vi "Protocol.Output Messages.vi"(8 "error in (no error)":errorcluster, 11 "J1939 Main Configuration":T1 {"Stream Refs"."Port Settings"."FD ISO Mode" items=["ISO", "Non ISO", "ISO Legacy"]; "Stream Refs"."Port Settings"."Termination" items=["Off", "On"]; "Stream Refs"."Port Settings"."Mode" items=["CAN 2.0", "CAN FD", "CAN FD+BRS"]}) -> (0 "error out":errorcluster)   [LabVIEW 2023, in "J1939 Addon Engine.lvlib"]
uses:
  J1939 Addon Engine.lvlib
  Types/Protocol.Configuration.ctl
  <vilib>/NI/NI VeriStand Addon Network Comm/Engine/VeriStand Comm.lvclass
  <vilib>/NI/NIVS Inline Async API/_VS Inline Async API/Process/Process.lvclass
  Types/Protocol.Refs.ctl
  Support Libraries/J1939 Utilities/Types/CAN Outgoing Message Cluster.ctl
  Types/Protocol.RQST Lookup Table Reference.ctl
  Types/Protocol.Address Table Reference.ctl
  Types/Protocol.XNET Settings.ctl
  <vilib>/NI/NIVS Inline Async API/_Data Access Engine/Data Access Engine/Types/Read.DVR.ctl
  <vilib>/NI/NIVS Inline Async API/_Data Access Engine/Access Type Classes/Read/Read.lvclass
  <vilib>/NI/NIVS Inline Async API/_Data Access Engine/Data Access Engine/Types/Write.DVR.ctl
  <vilib>/NI/NIVS Inline Async API/_Data Access Engine/Access Type Classes/Write/Write.lvclass
  Types/CounterAndProtectionFrames.ctl
  SubModules/Frame-Protection-Support/Source/Engine/Types/RT Frame Settings.ctl
  SubModules/Frame-Protection-Support/Source/Shared/Types/Exported Frame Type.ctl
  SubModules/Frame-Protection-Support/Source/Engine/Types/RT Protection Configuration.ctl
  SubModules/Frame-Protection-Support/Source/Shared/Types/Protection Type.ctl
  SubModules/Frame-Protection-Support/Source/Shared/Types/XNET Signal Configuration.ctl
  SubModules/Frame-Protection-Support/Source/Shared/Types/Exported Counter Settings.ctl
  SubModules/Frame-Protection-Support/Source/Shared/Types/Exported Event Trigger Type.ctl
  SubModules/CAN-Streaming-Support/Source/Addon/Addon Engine/Types/Engine Stream Refs.ctl
  SubModules/CAN-Streaming-Support/Source/Addon/Addon Shared/Types/Direction Filter.ctl
  SubModules/CAN-Streaming-Support/Source/Addon/Addon Shared/Types/Type Filter.ctl
  SubModules/CAN-Streaming-Support/Source/Addon/Addon Shared/Types/Filter Parameters.ctl
  SubModules/CAN-Streaming-Support/Source/Addon/Addon Engine/Types/Engine Stream Port Settings.ctl
  <vilib>/Platform/TimedLoop/XDataNode/timing_clust.ctl
  <vilib>/Platform/TimedLoop/XDataNode/nitl_modes.ctl
  <vilib>/Platform/TimedLoop/XDataNode/wakeup.ctl
  <vilib>/NI/NIVS Inline Async API/_Data Access Engine/Access Type Classes/Read/Read.lvclass/Read.ctl
  <vilib>/NI/NIVS Inline Async API/_Data Access Engine/Access Type Classes/Write/Write.lvclass/Write.ctl
  <vilib>/NI/NIVS Inline Async API/_VS Inline Async API/Process/Process.lvclass/Process.ctl
  <vilib>/NI/NIVS Inline Async API/_VS Inline Async API/Error Handling Process/SubVIs/Error.ConvertArray.vi
  <vilib>/NI/NIVS Inline Async API/_Data Access Engine/Data Access Engine/Methods/Data.Processes.Execute.vi
  <vilib>/NI/NIVS Inline Async API/_Data Access Engine/Data Access Engine/Methods/Read.Data.Detect.vi
  <vilib>/NI/NIVS Inline Async API/_Data Access Engine/Data Access Engine/Methods/Read.Data.vi
  SubModules/Frame-Protection-Support/Source/Engine/SubVIs/Determine Transmit.vi
  SubModules/Frame-Protection-Support/Source/Engine/SubVIs/Update Counter Signals.vi
  SubModules/Frame-Protection-Support/Source/Engine/SubVIs/Get Frame Data.vi
  SubModules/Frame-Protection-Support/Source/Engine/SubVIs/Convert EU Data to XNET Frame.vi
  SubModules/Frame-Protection-Support/Source/Engine/SubVIs/Update Protection Signals.vi
  SubModules/Frame-Protection-Support/Source/Engine/SubVIs/Determine Disabled.vi
  <vilib>/NI/NIVS Inline Async API/_Data Access Engine/Data Access Engine/Methods/Write.Data.Commit.vi
  <vilib>/NI/NIVS Inline Async API/_Data Access Engine/Access Type Classes/Read/Read.ProcessData.Detect.vi
  <vilib>/NI/NIVS Inline Async API/_Data Access Engine/Access Type Classes/Read/Read.ProcessData.vi
  SubModules/Frame-Protection-Support/Source/Engine/SubVIs/Determine Transmission.vi
  SubModules/Frame-Protection-Support/Source/Engine/SubVIs/Determine Periodic.vi
  SubModules/Frame-Protection-Support/Source/Engine/SubVIs/Set Counter Signal.vi
  SubModules/Frame-Protection-Support/Source/Engine/SubVIs/Calculate Counter Value.vi
  SubModules/Frame-Protection-Support/Source/Engine/SubVIs/Set Protection Signal.vi
  SubModules/Frame-Protection-Support/Source/Engine/SubVIs/Calculate Protection Value.vi
  <vilib>/NI/NIVS Inline Async API/_Data Access Engine/Access Type Classes/Write/Write.Commit.vi
  <vilib>/NI/NIVS Inline Async API/_Data Access Engine/Data Access Engine/Methods/Write.Data.Buffer.vi
  SubModules/Frame-Protection-Support/Source/Engine/SubVIs/Get Protection Signals.vi
  <vilib>/NI/NIVS Inline Async API/_Data Access Engine/Access Type Classes/Write/Write.Buffer.vi
  <vilib>/xnet/xnet.llb/XNET Convert.vi
  <vilib>/xnet/xnet.llb/XNET Convert (Signal to Frame Raw).vi
  <vilib>/xnet/xnet.llb/XNET Convert (Signal to Frame CAN).vi
  <vilib>/xnet/xnet.llb/XNET Write (Frame CAN).vi
  <vilib>/Platform/TimedLoop/XDataNode/XDataNode.xnode
  SubModules/Frame-Protection-Support/Source/Engine/Protection and Counter Support Engine.lvlib
  <vilib>/Platform/TimedLoop/XDataNode/XDNodeRunTimeDep.lvlib
  Support Libraries/J1939 Utilities/J1939 Utilities.lvlib
  <vilib>/NI/NIVS Inline Async API/_Data Access Engine/Data Access Engine/Data Access Engine.lvclass
  SubModules/Frame-Protection-Support/Source/Shared/Protection and Counter Support Shared.lvlib
  SubModules/CAN-Streaming-Support/Source/Addon/Addon Shared/CAN Stream Support Shared.lvlib
  SubModules/CAN-Streaming-Support/Source/Addon/Addon Engine/CAN Stream Support Engine.lvlib
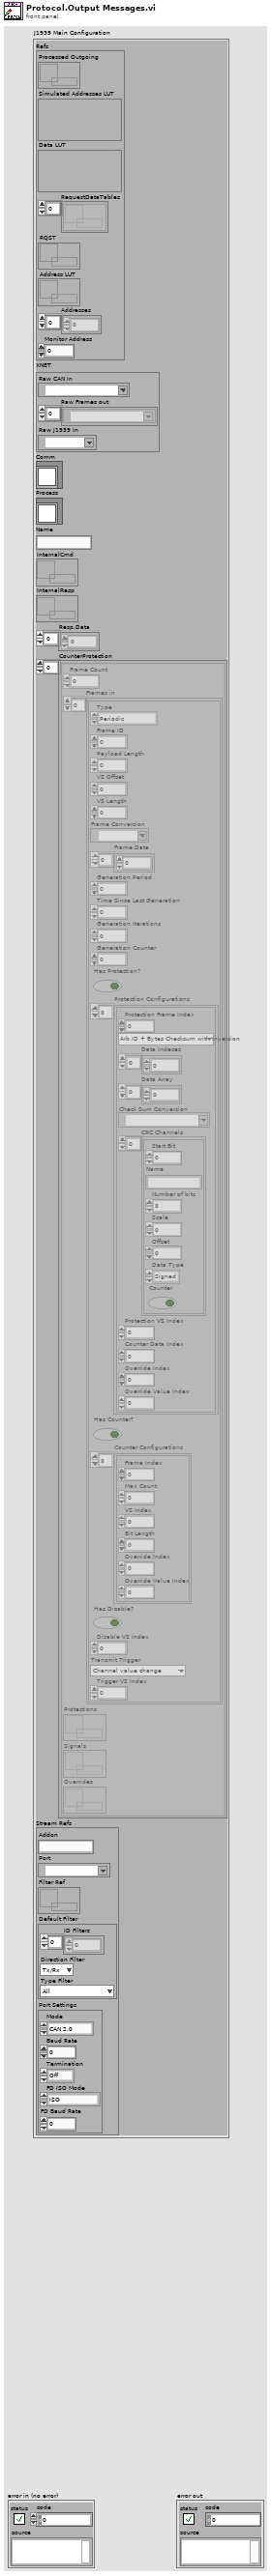
[diagram p1: front panel]
types:
  T1 = typedef "J1939 Addon Engine.lvlib/Protocol.Configuration.ctl" = cluster{"Refs":T2, "XNET":T5, "Comm":refnum<class "VeriStand Comm.lvclass">, "Process":refnum<class "Process.lvclass">, "Name":string, "InternalCmd":T6, "InternalResp":T7, "Resp.Data":dbl[], "CounterProtection":T8[], "Stream Refs":T16}
  T2 = typedef "J1939 Addon Engine.lvlib/Protocol.Refs.ctl" = cluster{"Processed Outgoing":refnum<queue>, "Simulated Addresses LUT":variant, "Data LUT":variant, "RequestDataTables":refnum<k33>[], "RQST":T3, "Address LUT":T4, "Addresses":u8[], "Monitor Address":u8}
  T3 = typedef "J1939 Addon Engine.lvlib/Protocol.RQST Lookup Table Reference.ctl" = refnum<data-value>
  T4 = typedef "J1939 Addon Engine.lvlib/Protocol.Address Table Reference.ctl" = refnum<data-value>
  T5 = typedef "J1939 Addon Engine.lvlib/Protocol.XNET Settings.ctl" = cluster{"Raw CAN In":refnum<k21>, "Raw Frames out":refnum<k21>[], "Raw J1939 In":refnum<k21>}
  T6 = typedef "Data Access Engine.lvlib/Data Access Engine.lvclass/Read.DVR.ctl" = refnum<data-value>
  T7 = typedef "Data Access Engine.lvlib/Data Access Engine.lvclass/Write.DVR.ctl" = refnum<data-value>
  T8 = typedef "J1939 Addon Engine.lvlib/CounterAndProtectionFrames.ctl" = cluster{"Frame Count":i32, "Frames in":T9[], "Protections":T7, "Signals":T6, "Overrides":T6}
  T9 = typedef "Protection and Counter Support Engine.lvlib/RT Frame Settings.ctl" = cluster{"Type":T10, "Frame ID":u32, "Payload Length":u32, "VS Offset":i32, "VS Length":i32, "Frame Conversion":refnum<k21>, "Frame.Data":dbl[], "Generation Period":u32, "Time Since Last Generation":u32, "Generation Iterations":u32, "Generation Counter":u32, "Has Protection?":bool, "Protection Configurations":T11[], "Has Counter?":bool, "Counter Configurations":T14[], "Has Disable?":bool, "Disable VS Index":i32, "Transmit Trigger":T15, "Trigger VS Index":i32}
  T10 = typedef "Protection and Counter Support Shared.lvlib/Exported Frame Type.ctl" = enum16{"Periodic", "Event", "Periodic/Event"}
  T11 = typedef "Protection and Counter Support Engine.lvlib/RT Protection Configuration.ctl" = cluster{"Protection Frame Index":i32, "Protection Type":T12, "Data Indeces":i32[], "Data Array":dbl[], "Check Sum Conversion":refnum<k21>, "CRC Channels":T13[], "Protection VS Index":i32, "Counter Data Index":i32, "Override Index":i32, "Override Value Index":i32}
  T12 = typedef "Protection and Counter Support Shared.lvlib/Protection Type.ctl" = enum16{"Arb ID + Bytes Checksum with Inversion", "Arb ID + Bytes CRC with Inversion", "Reversed Raw Signal Checksum with Inversion", "Concatenated Two's Compliment"}
  T13 = typedef "Protection and Counter Support Shared.lvlib/XNET Signal Configuration.ctl" = cluster{"Start Bit":i32, "Name":string, "Number of bits":i32, "Scale":dbl, "Offset":dbl, "Data Type":u32, "Counter":bool}
  T14 = typedef "Protection and Counter Support Shared.lvlib/Exported Counter Settings.ctl" = cluster{"Frame Index":i32, "Max Count":dbl, "VS Index":i32, "Bit Length":i64, "Override Index":i32, "Override Value Index":i32}
  T15 = typedef "Protection and Counter Support Shared.lvlib/Exported Event Trigger Type.ctl" = enum16{"Channel value change", "Trigger channel (not zero)", "Channel value change or trigger channel (not zero)", "Trigger channel (any value change)", "Channel value change or trigger channel (any value change)"}
  T16 = typedef "CAN Stream Support Engine.lvlib/Engine Stream Refs.ctl" = cluster{"Addon":string, "Port":refnum<k21>, "Filter Ref":refnum<data-value>, "Default Filter":T17, "Port Settings":T20}
  T17 = typedef "CAN Stream Support Shared.lvlib/Filter Parameters.ctl" = cluster{"ID Filters":u32[], "Direction Filter":T18, "Type Filter":T19}
  T18 = typedef "CAN Stream Support Shared.lvlib/Direction Filter.ctl" = enum16{"Tx/Rx", "Rx", "Tx"}
  T19 = typedef "CAN Stream Support Shared.lvlib/Type Filter.ctl" = enum16{"All", "CAN Data", "CAN Remote", "CAN Bus Error", "CAN 2.0 Data", "CAN FD Data", "CAN FD+BRS Data", "J1939 Data", "Delay", "Log Trigger", "Start Trigger"}
  T20 = typedef "CAN Stream Support Engine.lvlib/Engine Stream Port Settings.ctl" = cluster{"Mode":u32, "Baud Rate":u64, "Termination":u32, "FD ISO Mode":u32, "FD Baud Rate":u64}
  T21 = typedef "XDNodeRunTimeDep.lvlib/timing_clust.ctl" = cluster{"Expected End [f-1]":u64, "Actual End [f-1]":u64, "Finished Late? [f-1]":bool, "Expected End [i-1]":u64, "Actual End [i-1]":u64, "Finished Late? [i-1]":bool, "Expected Start [i]":u64, "Actual Start [i]":u64, "Expected Start [f]":u64, "Actual Start [f]":u64, "Source Name":string, "Structure Name":string, "Period":i64, "Deadline":i64, "Offset":i64, "Start":i64, "Priority":i32, "Timeout":i32, "Mode":T22, "Wakeup Reason":T23, "Error":errorcluster, "Source Type":string, "Secondary Source Type":string, "Global End Time":u64, "Global Start Time":u64, "Frame Duration":u64, "Iteration Duration":u64, "Assigned CPU":i32, "I/O Scan Engine Mode":u32}
  T22 = typedef "XDNodeRunTimeDep.lvlib/nitl_modes.ctl" = enum32{"No Change", "Process missed periods, maintain original phase", "Discard missed periods, maintain original phase", "Process missed periods, ignore original phase", "Discard missed periods, ignore original phase"}
  T23 = typedef "XDNodeRunTimeDep.lvlib/wakeup.ctl" = enum32{"Normal", "Aborted", "Asynchronous wakeup", "Timing source error", "Timed loop error", "Timeout"}
  T24 = typedef "XNET Frame CAN.ctl" = cluster{"timestamp":timestamp, "payload":u8[], "identifier":u32, "type":T25, "extended?":bool, "echo?":bool}
  T25 = typedef "XNET Frame Type CAN.ctl" = u8
  T26 = typedef "J1939 Utilities.lvlib/CAN Outgoing Message Cluster.ctl" = cluster{"Identifier":u32, "Data":u8[]}
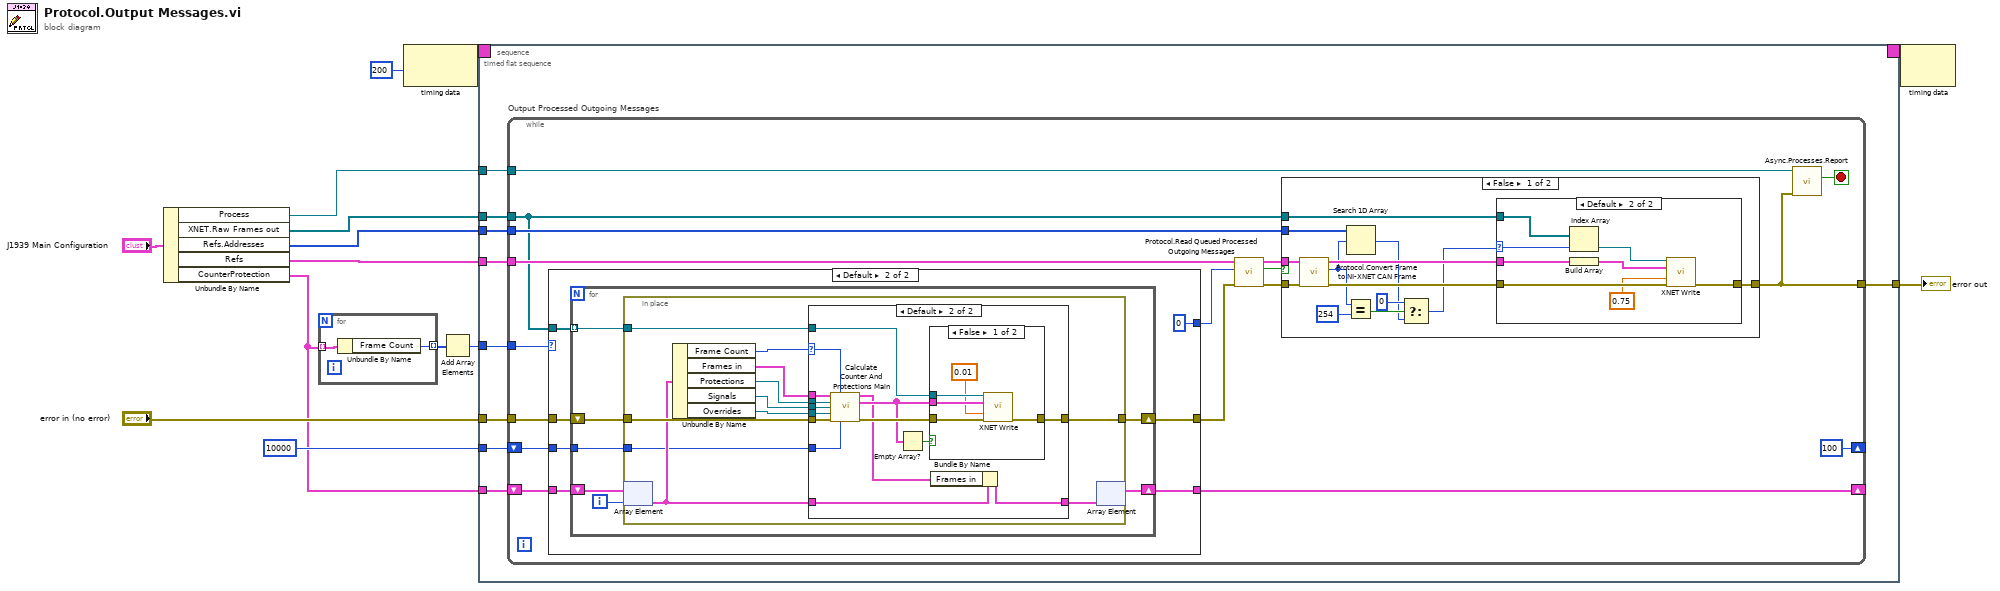
[diagram p0: block diagram]
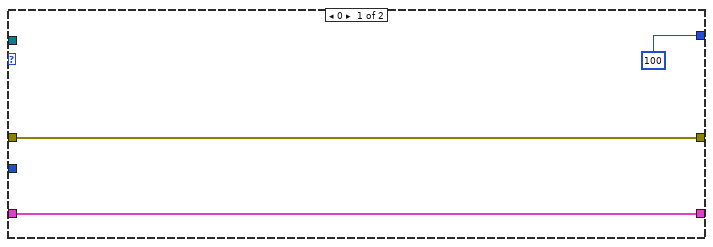
[diagram p2: hidden frame]
diagram:
  n1 = Unbundle By Name("J1939 Main Configuration") -> ("Process"=w14:refnum<class "Process.lvclass">, "XNET.Raw Frames out"=w13:refnum<k21>[], "Refs.Addresses"=w8:u8[], "Refs"=w12:T2, "CounterProtection"=w3:T8[])
  n2 = for {
    tunnel: w3 -> [w16] mode=indexing
    tunnel: [w15] -> w2 mode=indexing
    n3 = Unbundle By Name(w16) -> ("Frame Count"=w15:i32)
  }
  n4 = node-c288(200 ("Priority")) -> (w7:T21)
  n5 = Add Array Elements(numeric array=w2) -> (sum=w1:i32)
  n6 = timed-sequence {
    timing: w7 -> [_]
    timing-out: [_] -> w6
    tunnel: w14 -> [w25]
    tunnel: w13 -> [w24]
    tunnel: w12 -> [w23]
    tunnel: "error in (no error)" -> [w22]
    tunnel: [w21] -> w9
    tunnel: w8 -> [w20]
    tunnel: w3 -> [w19]
    tunnel: 10000 -> [w18]
    tunnel: w1 -> [w17]
    n7 = timed-flat-sequence {
      tunnel: w25 -> [w34]
      tunnel: w24 -> [w33]
      tunnel: w23 -> [w32]
      tunnel: w22 -> [w31]
      tunnel: [w30] -> w21
      tunnel: w20 -> [w29]
      tunnel: w19 -> [w28]
      tunnel: w18 -> [w27]
      tunnel: w17 -> [w26]
      n8 = while "Output Processed Outgoing Messages" {
        tunnel: w32 -> [w51]
        tunnel: w31 -> [w41]
        tunnel: [w42] -> w30
        tunnel: w33 -> [w39]
        tunnel: w34 -> [w45]
        tunnel: w29 -> [w47]
        shift-right: [w43] -> _
        shift-left: w28 -> [w44]
        shift-right: [100] -> _
        shift-left: w27 -> [w38]
        tunnel: w26 -> [w36]
        stop <- w46 stop-if-true
        n9 = case shown="Default" w36 {
          tunnel: w44 -> [w54 w61]
          tunnel: [w54 w60] -> w43
          tunnel: w41 -> [w53 w59]
          tunnel: [w53 w58] -> w40
          tunnel: w39 -> [_ w57]
          tunnel: w38 -> [_ w56]
          tunnel: [100 ("timeout in ms (-1)") 0 ("timeout in ms (-1)")] -> w35
          frame 0 {
          }
          frame Default {
            n10 = for {
              shift-right: [w67] -> w58
              shift-left: w59 -> [w68]
              tunnel: w57 -> [w66] mode=indexing
              shift-right: [w63] -> w60
              shift-left: w61 -> [w64]
              tunnel: w56 -> [w62]
              i -> [w65]
              n11 = in-place {
                in-place-border: w68 -> [w79]
                in-place-border: [w78] -> w67
                in-place-border: w66 -> [w77]
                in-place-border: w62 -> [w70]
                n12 = in-place-array #1(w64, w65) -> (w73:T8)
                n13 = Unbundle By Name(w73) -> ("Frame Count"=w71:i32, "Frames in"=w76:T9[], "Protections"=w75:T7, "Signals"=w74:T6, "Overrides"=w69:T6)
                n14 = case shown="Default" w71 {
                  selector: w71 -> [_ w84]
                  tunnel: w79 -> [w81 w96]
                  tunnel: [w81 w95] -> w78
                  tunnel: w77 -> [_ w94]
                  tunnel: w76 -> [_ w90]
                  tunnel: w75 -> [_ w89]
                  tunnel: w74 -> [_ w88]
                  tunnel: w73 -> [w80 w87]
                  tunnel: [w80 w85] -> w72
                  tunnel: w70 -> [_ w83]
                  tunnel: w69 -> [_ w82]
                  frame 0 {
                  }
                  frame Default {
                    n15 = call "Calculate Counter And Protections Main.vi"("Frames in"=w90, "Frame Count"=w84, "Protections"=w89, "Signals"=w88, "Overrides"=w82, "error in (no error)"=w96, "timeout ms"=w83) -> ("Frames out"=w86:T9[], "Frames"=w92:T24[], "error out"=w93:errorcluster)  [unwired: 5 in, 1 out]
                    n16 = Empty Array?(array=w92) -> (empty?=w91:bool)
                    n17 = case shown="False" w91 {
                      tunnel: [w101 w102] -> w95
                      tunnel: w94 -> [w100 _]
                      tunnel: w93 -> [w99 w102]
                      tunnel: w92 -> [w98 _]
                      frame False {
                        n18 = call-poly <vilib>:"XNET Write.vi"("session in"=w100, "data"=w98, "timeout (10)"=0.01, "error in (no error)"=w99) -> ("error out"=w101:errorcluster)  [unwired: 11 out]
                      }
                      frame True {
                      }
                    }
                    n19 = Bundle By Name(cluster=w87, "Frames in"=w86) -> (w85:T8)
                  }
                }
                n20 = in-place-array #1(w72) -> (w63:T8[])  [unwired: 1 out]
              }
            }
          }
        }
        n21 = call "Protocol.Read Queued Processed Outgoing Messages.vi"("error in (no error)"=w40, "timeout in ms (-1)"=w35, "J1939 Cluster"=w51) -> ("error out"=w50:errorcluster, "timed out?"=w48:bool, "Frame"=w49:T26)  [unwired: 6 in]
        n22 = case shown="False" w48 {
          tunnel: w50 -> [w103 w125]
          tunnel: w49 -> [w115 _]
          tunnel: w39 -> [w110 _]
          tunnel: [w114 w125] -> w42
          tunnel: w47 -> [w111 _]
          frame False {
            n23 = call "Protocol.Convert Frame to NI-XNET CAN Frame.vi"("error in (no error)"=w103, "Data to Send"=w115) -> ("error out"=w112:errorcluster, "Source Address"=w105:u8, "CAN frame"=w113:T24)  [unwired: 7 out]
            n24 = Search 1D Array(1D array=w111, element=w105) -> (index of element=w104:i32)  [unwired: 1 in]
            n25 = Equal?(x=w105, y=u8 254) -> (x = y?=w108:bool)
            n26 = Select(t=0, s=w108, f=w104) -> (s? t:f=w106:i32)
            n27 = case shown="Default" w106 {
              selector: w106 -> [_ w119]
              tunnel: [w116 w124] -> w114
              tunnel: w113 -> [_ w123]
              tunnel: w112 -> [w116 w122]
              tunnel: w110 -> [_ w117]
              frame -1 {
              }
              frame Default {
                n28 = Index Array(array=w117, index=w119) -> (element=w120:refnum<k21>)
                n29 = Build Array(w123) -> (w118:T24[])
                n30 = call-poly <vilib>:"XNET Write.vi"("session in"=w120, "data"=w118, "timeout (10)"=0.75, "error in (no error)"=w122) -> ("error out"=w124:errorcluster)  [unwired: 11 out]
              }
            }
          }
          frame True {
          }
        }
        n31 = call <vilib>:"Async.Processes.Report.vi"("Error"=w42, "Process in"=w45) -> ("Stop"=w46:bool)  [unwired: 8 in, 1 out]
      }
    }
  }
  "error out" <- w9
  n32 = node-c288(w6) -> ()  [unwired: 1 out]
